vi "Create Logger.vi"(4 "Old Files Configuration":T1={"Action on Max Folder Size"=enum."Remove Oldest Files", "Max # Files in Folder"=10}, 6 "Multiple Files Configuration":T3={"Multiple Files Action"=enum."Seperate based on size", "Max File Size (MB)"=100.0, "Max Time in File (s)"=3600.0}, 8 "Error In":errorcluster, 10 "Base Folder":path caption="Base Folder (dialog)", 11 "Base File Name":string="Data") -> (0 "Error Out":errorcluster, 2 "Final Path":path, 3 "TDMS Log Out":refnum<class "TDMS Logger.lvclass">)   [LabVIEW 2015, in "TDMS Logger.lvlib" / "TDMS Logger.lvclass"]
doc: "Create and run the asynchronous TDMS logger.\n\n<b>Base File Name</b> - here you specify the base for the name of the file that will be used by this data logger. This base name will get an appendix with current date and time or number depending on the multiple files configuration.\n\n<b>Base Folder</b> - this input defines the path that will be used to store your logged TDMS files. If you do not wire anything a dialog will be shown. If the path is invalid the default path will be used: Application Directory/Data Folder\n\n<b>Multiple Files Configuration</b> - specify if you want to create multiple TDMS files from your data or not. Also define what should be the maximum size for the files if you chose the size based option or the maximum time spent in one file if you chose the time based option.\n\n<b>Old Files Configuration</b> - choose if you want to delete old files or not. Specify maximum number of files in this folder with the name containing <b>Base File Name</b>\n\n<b>Final Path</b> - this output can be used to check what is the final folder path used by the logger."
uses:
  TDMS Logger.lvclass
  _Typedefs/Multiple Files Configuration.ctl
  _Typedefs/Multiple Files Action.ctl
  _Typedefs/Old Files Configuration.ctl
  _Typedefs/Folder Size Limit Reached.ctl
  TDMS Logger.lvclass/TDMS Logger.ctl
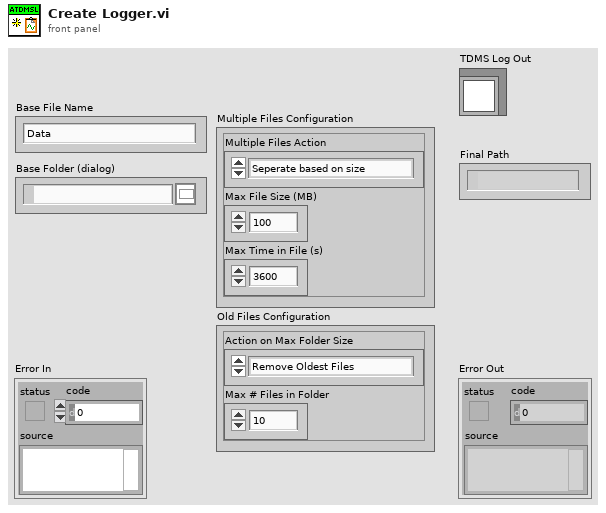
[diagram p1: front panel]
types:
  T1 = typedef "TDMS Logger.lvlib/TDMS Logger.lvclass/Old Files Configuration.ctl" = cluster{"Action on Max Folder Size":T2, "Max # Files in Folder":i32}
  T2 = typedef "TDMS Logger.lvlib/TDMS Logger.lvclass/Folder Size Limit Reached.ctl" = enum16{"Do Nothing", "Remove Oldest Files"}
  T3 = typedef "TDMS Logger.lvlib/TDMS Logger.lvclass/Multiple Files Configuration.ctl" = cluster{"Multiple Files Action":T4, "Max File Size (MB)":dbl, "Max Time in File (s)":dbl}
  T4 = typedef "TDMS Logger.lvlib/TDMS Logger.lvclass/Multiple Files Action.ctl" = enum16{"Seperate based on size", "Seperate based on time", "Single file"}
  T5 = typedef "TDMS Logger.lvlib/TDMS Logger.lvclass/Data Queues.ctl" = cluster{"Single Queue":refnum<queue>, "Double Queue":refnum<queue>, "U8 Queue":refnum<queue>, "U16 Queue":refnum<queue>, "String Queue":refnum<queue>, "Waveform Queue":refnum<queue>, "I8 Queue":refnum<queue>, "I16 Queue":refnum<queue>}
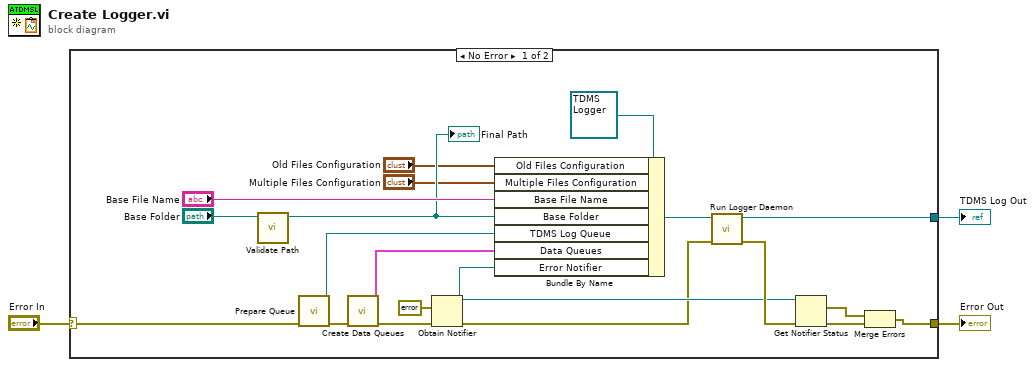
[diagram p0: block diagram]
diagram:
  n1 = case shown="No Error" "Error In" {
    selector: "Error In" -> [w22 w24]
    tunnel: [w12 w24] -> w2
    tunnel: [w18 _] -> w1
    frame No Error {
      n2 = call "Validate Path.vi"("Base Folder"="Base Folder") -> ("Valid Path"=w19:path)  [unwired: 10 in]
      "Final Path" <- w19
      n3 = call "Prepare Queue.vi"("Error In"=w22) -> ("Error Out"=w6:errorcluster, "TDMS Log Queue"=w17:refnum<queue>)  [unwired: 9 in]
      n4 = call "Create Data Queues.vi"("Error In"=w6) -> ("Error Out"=w5:errorcluster, "Data Queues"=w8:T5)  [unwired: 9 in]
      n5 = Obtain Notifier(notification data type=errorcluster {"status"=FALSE, "code"=0, "source"=""} ("Logger Error"), error in (no error)=w5) -> (notifier out=w7:refnum<notifier>, error out=w4:errorcluster)  [unwired: 2 in, 1 out]
      n6 = Bundle By Name(cluster=refnum<class "TDMS Logger.lvclass"> refnum ("TDMS Log in"), "Old Files Configuration"="Old Files Configuration", "Multiple Files Configuration"="Multiple Files Configuration", "Base File Name"="Base File Name", "Base Folder"=w19, "TDMS Log Queue"=w17, "Data Queues"=w8, "Error Notifier"=w7) -> (w21:refnum<class "TDMS Logger.lvclass">)
      n7 = call "Run Logger Daemon.vi"("Error In"=w4, "TDMS Log In"=w21) -> ("Error Out"=w15:errorcluster, "TDMS Log Out"=w18:refnum<class "TDMS Logger.lvclass">)  [unwired: 8 in]
      n8 = Get Notifier Status(notifier=w7, error in (no error)=w15) -> (current notification=w13:errorcluster, error out=w14:errorcluster)  [unwired: 3 out]
      n9 = Merge Errors(w13, w14) -> (w12:errorcluster)
    }
    frame Error {
    }
  }
  "Error Out" <- w2
  "TDMS Log Out" <- w1
